vi "BiFuncHelp_MatrixPlus.vi"(9 "B":T1, 10 "A":T1, 11 "Variant":variant) -> (0 "Error":bool, 3 "Output":T1)   [LabVIEW 2019, in "Trajectory_Library.lvlib"]
uses:
  Trajectory_Library.lvlib
  <vilib>/Analysis/Matrix/Datatypes/RealMatrix.ctl
  <vilib>/Analysis/Matrix/Numeric/Add/Add - RM,RM.vi
  <vilib>/Analysis/Matrix/NI_Matrix.lvlib
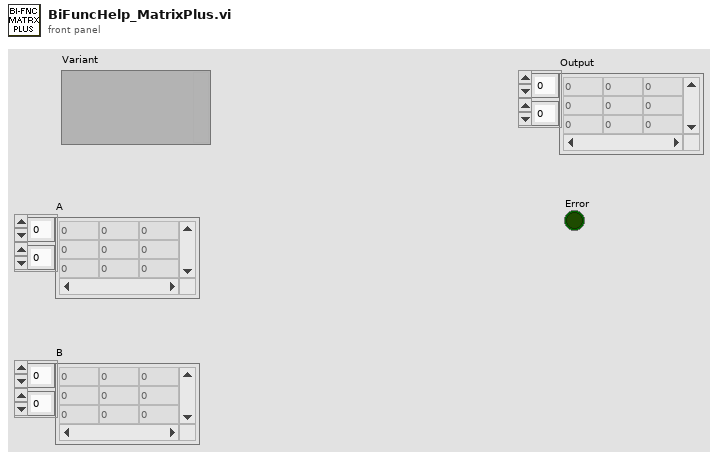
[diagram p1: front panel]
types:
  T1 = typedef "NI_Matrix.lvlib/RealMatrix.ctl" = dbl[][]
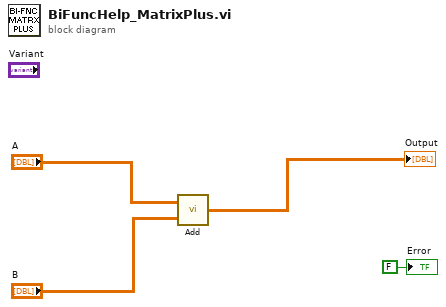
[diagram p0: block diagram]
diagram:
  n1 = call-poly <vilib>:"Add.vi"("Real Matrix B"="B", "Real Matrix A"="A") -> ("A + B"=→"Output":T1)
  "Error" <- FALSE ("Error")
